vi "5006 Unexpected Control Class.vi"(8 "error in (no error)":errorcluster, 10 "Expected Classes":string, 11 "Class Name":string) -> (0 "error out":errorcluster)   [LabVIEW 2020, in "MacroAssert.lvlib" / "Custom Errors.lvlib"]
uses:
  Custom Errors.lvlib
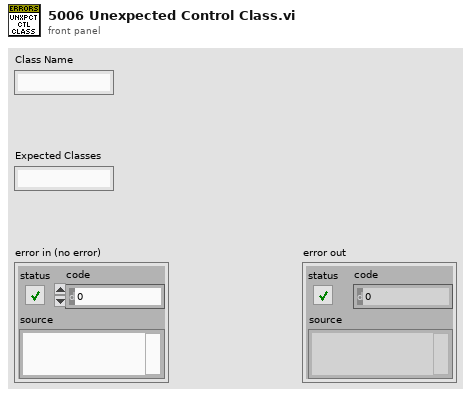
[diagram p1: front panel]
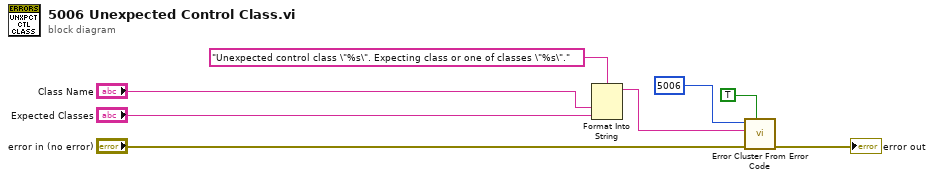
[diagram p0: block diagram]
diagram:
  n1 = Format Into String(format string="Unexpected control class \"%s\". Expecting class or one of classes \"%s\".", "Class Name", "Expected Classes") -> (resulting string=w4:string)  [unwired: 2 in, 1 out]
  n2 = call <vilib>:"Error Cluster From Error Code.vi"("show call chain? (False)"=TRUE, "error in (no error)"="error in (no error)", "error message (\"\")"=w4, "error code (0)"=5006) -> ("error out"=→"error out":errorcluster)  [unwired: 5 in]
